vi "longitude.vi"() -> ()   [LabVIEW 2015, in "Biblioteka moduł map v3.lvlib" / "Zmienne globalne.lvlib"]
uses:
  Zmienne globalne.lvlib
panel:
  in  "Longitude":dbl
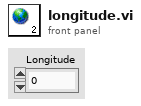
[diagram p1: front panel]
diagram:
